vi "Construct Terminal Visibility Binding.vi"(7 "Initial Visible State (T)":bool=TRUE, 9 "Inverse Visible Logic? (F)":bool, 10 "Ctl Refnum":refnum<vi>) -> (0 "error out":errorcluster, 3 "TerminalVisibilityBinding":refnum<class "TerminalVisibilityBinding.lvclass">)   [LabVIEW 2020, in "TerminalVisibilityBinding.lvclass"]
doc: "构建终端可见性绑定"
uses:
  TerminalVisibilityBinding.lvclass
  TerminalPropertyBinding/TerminalPropertyBinding.lvclass/TerminalPropertyBinding.ctl
  TerminalVisibilityBinding.lvclass/TerminalVisibilityBinding.ctl
  TerminalPropertyBinding/TerminalPropertyBinding.lvclass
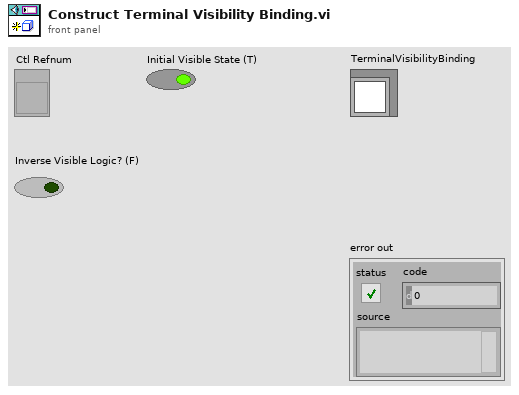
[diagram p1: front panel]
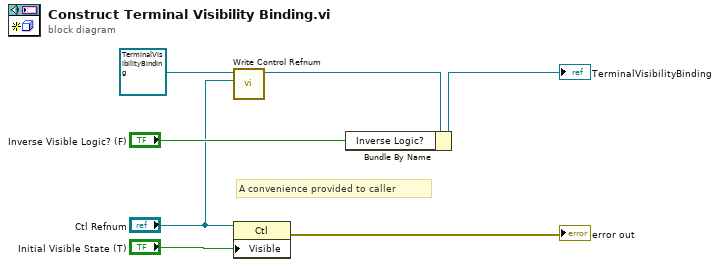
[diagram p0: block diagram]
diagram:
  # "A convenience provided to caller"
  n1 = call "Write Control Refnum.vi"("Ctl Refnum"="Ctl Refnum", "TerminalReference in"=refnum<class "TerminalVisibilityBinding.lvclass"> refnum ("TerminalVisibilityBinding")) -> ("TerminalReferenceBinding Out"=w2:refnum<class "TerminalVisibilityBinding.lvclass">)  [unwired: 9 in]
  n2 = property class="Ctl"(reference="Ctl Refnum", "Visible"="Initial Visible State (T)") -> (error out=→"error out":errorcluster)  [unwired: 1 in, 1 out]
  n3 = Bundle By Name(cluster=w2, "Inverse Logic?"="Inverse Visible Logic? (F)") -> (→"TerminalVisibilityBinding":refnum<class "TerminalVisibilityBinding.lvclass">)
